vi "VIP Message.vi"(5 "Latest VIP":T1, 8 "Latest Version":string, 9 "Current Version":string) -> (3 "Continue":bool)   [LabVIEW 2014, in "Raspberry Pi Compatible Compiler for LabVIEW.lvlib"]
uses:
  Raspberry Pi Compatible Compiler for LabVIEW.lvlib
  System.Windows.Forms
  GitHub/TypeDefs/GitHubContents_TD.ctl
  Messaging/SimpleMessaging.lvlib
  GitHub/GitHub API.lvlib
panel:
  out "Animated Image":i16(ring) caption="Ring 2"
  out "Message":string
  in  "WebBrowser":refnum<k24>(container)
  in  "Compile":bool
  in  "Don't Continue":bool
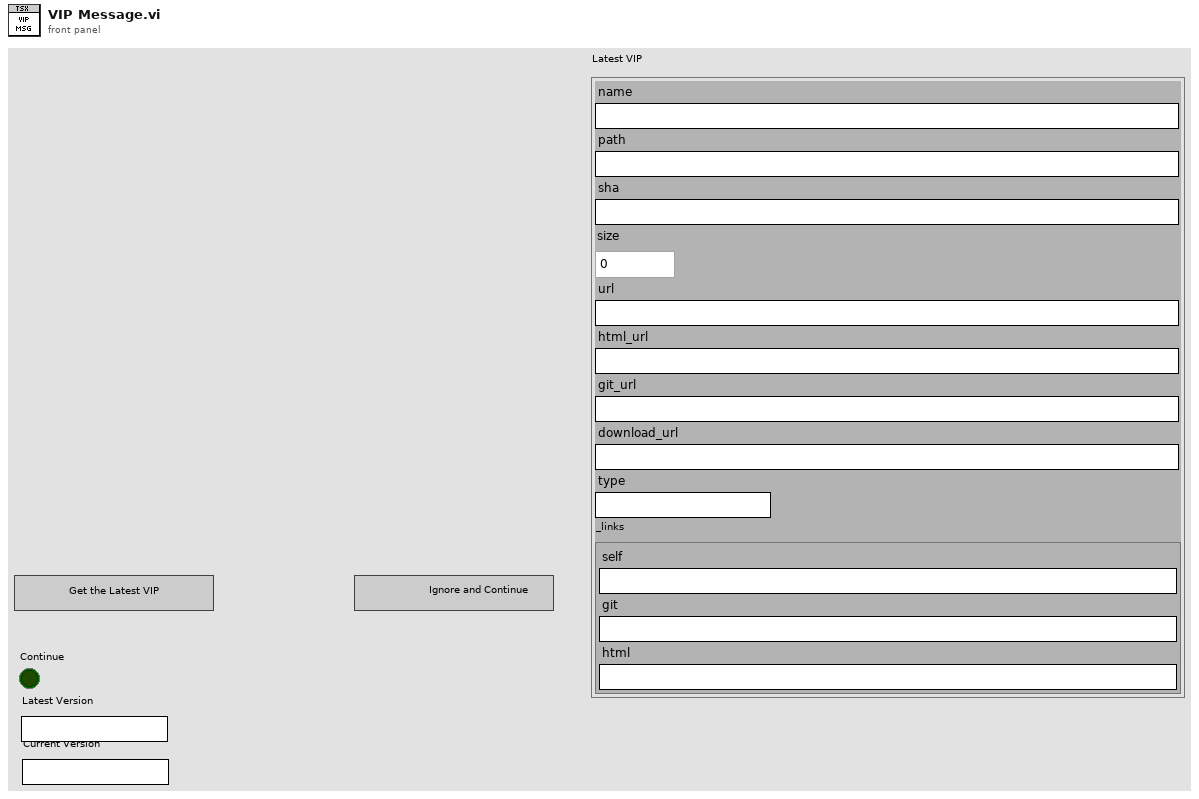
[diagram p1: front panel]
types:
  T1 = typedef "Raspberry Pi Compatible Compiler for LabVIEW.lvlib/GitHub API.lvlib/GitHubContents_TD.ctl" = cluster{"name":string, "path":string, "sha":string, "size":dbl, "url":string, "html_url":string, "git_url":string, "download_url":string, "type":string, "_links":cluster{"self":string, "git":string, "html":string}}
  T2 = typedef "Raspberry Pi Compatible Compiler for LabVIEW.lvlib/SimpleMessaging.lvlib/MessageQueueTD.ctl" = refnum<queue>
  T3 = enum32{"Invalid", "Standard", "Closed", "Hidden", "Minimized", "Maximized"}
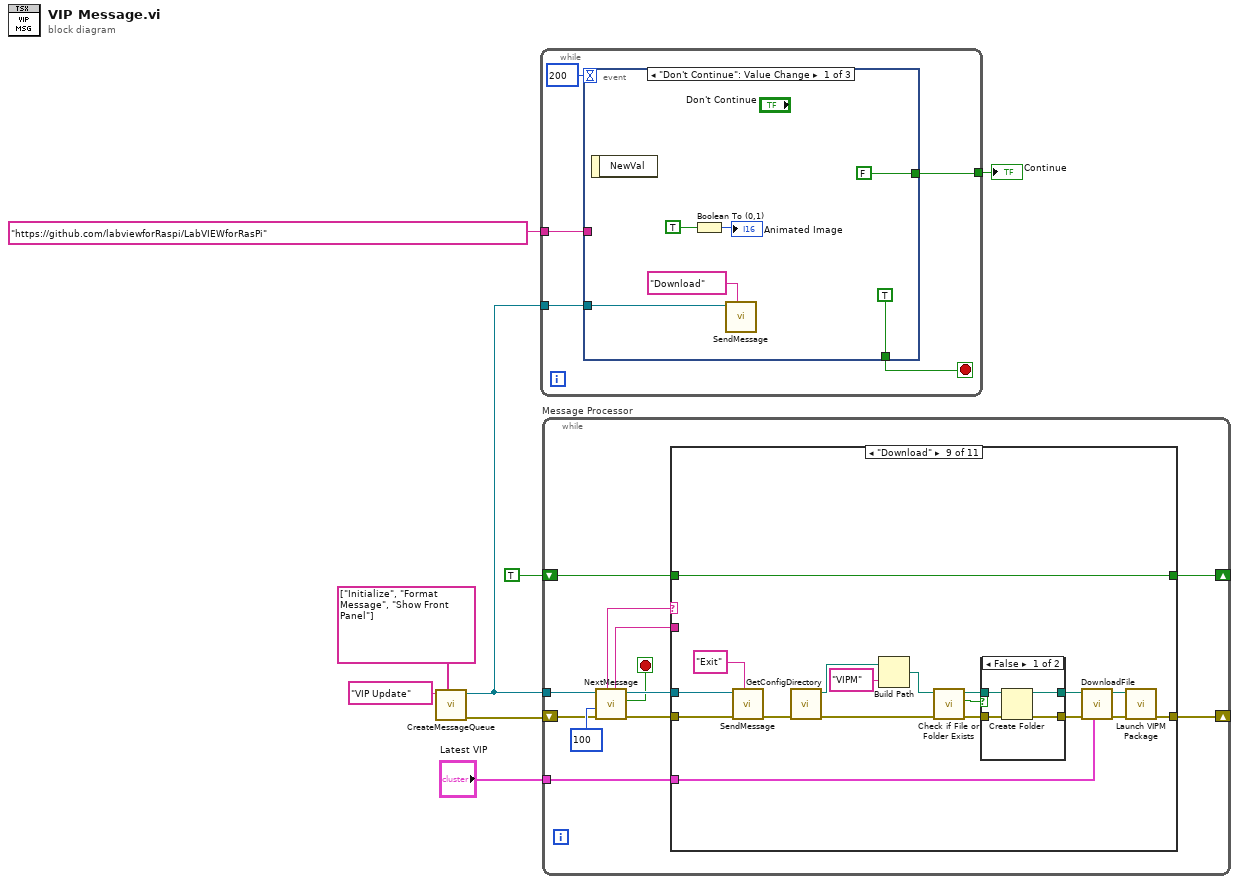
[diagram p0: block diagram]
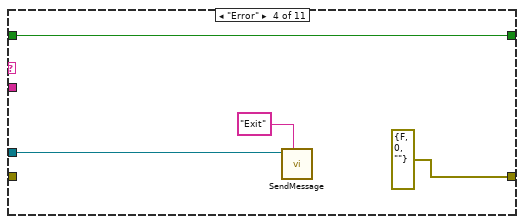
[diagram p5: hidden frame]
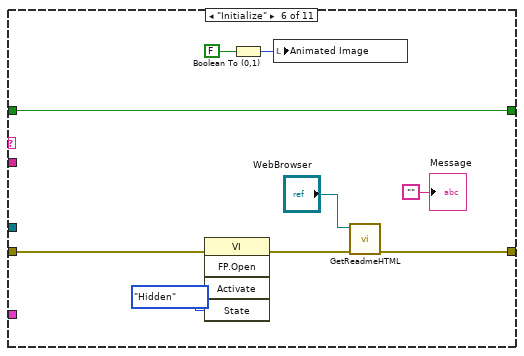
[diagram p7: hidden frame]
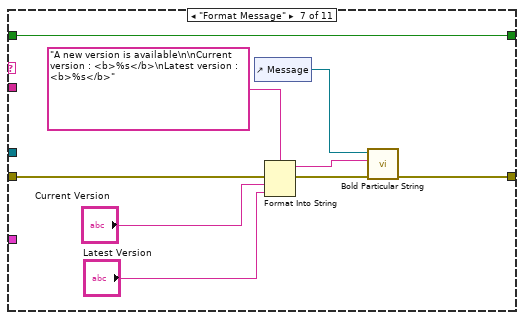
[diagram p8: hidden frame]
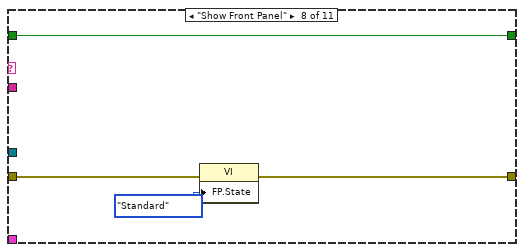
[diagram p9: hidden frame]
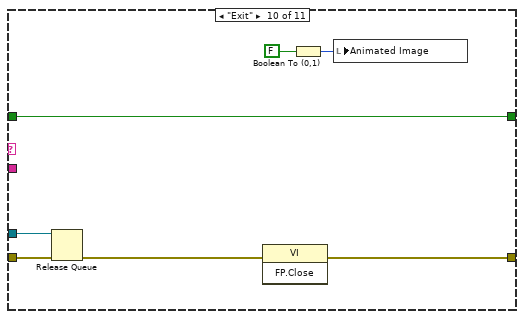
[diagram p11: hidden frame]
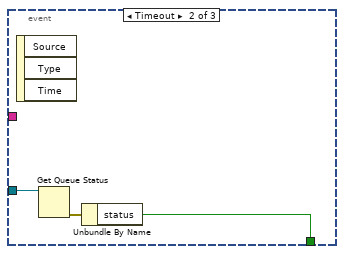
[diagram p13: hidden frame]
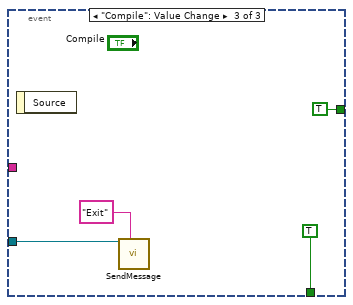
[diagram p14: hidden frame]
diagram:
  n1 = call "CreateMessageQueue.vi"("initial message names"=string[] ["Initialize", "Format Message", "Show Front Panel"], "message queue name"="VIP Update" ("name (unnamed)")) -> ("error out"=w2:errorcluster, "message queue out"=w3:T2)  [unwired: 5 in, 1 out]
  n2 = while {
    tunnel: "https://github.com/labviewforRaspi/LabVIEWforRasPi" ("URL") -> [w13]
    tunnel: [w12] -> w7
    tunnel: w3 -> [w10]
    stop <- w11 stop-if-true
    n3 = event shown="[0] \"Don't Continue\": Value Change" {
      selector: _ -> [_ _ _]
      dyn-events: _ -> [_ _ _]
      timeout: 200 -> [_ _ _]
      tunnel: w13 -> [_ _ _]
      tunnel: [TRUE w20 TRUE] -> w11
      tunnel: [FALSE _ TRUE] -> w12
      tunnel: w10 -> [w17 w22 w24]
      event "Don't Continue": Value Change {
        n4 = event-data() -> ()  [unwired: 1 in, 1 out]
        n5 = Boolean To (0,1)(Boolean=TRUE) -> (0, 1=→"Animated Image":i16)
        n6 = call "SendMessage.vi"("Name"="Download" ("Command"), "message queue in"=w17) -> ()  [unwired: 5 in, 3 out]
      }
      event Timeout {
        n7 = event-data() -> ()  [unwired: 1 in, 3 out]
        n8 = Get Queue Status(queue=w22) -> (error out=w21:errorcluster)  [unwired: 2 in, 7 out]
        n9 = Unbundle By Name(w21) -> ("status"=w20:bool)
      }
      event "Compile": Value Change {
        n10 = event-data() -> ()  [unwired: 1 in, 1 out]
        n11 = call "SendMessage.vi"("Name"="Exit", "message queue in"=w24) -> ()  [unwired: 5 in, 3 out]
      }
    }
  }
  "Continue" <- w7
  n12 = while "Message Processor" {
    shift-left: w2 -> [w29]
    shift-right: [w36] -> _
    shift-left: TRUE -> [w38]
    shift-right: [w37] -> _
    tunnel: w3 -> [w30]
    tunnel: "Latest VIP" -> [w27]
    stop <- w28 stop-if-true
    n13 = call "NextMessage.vi"("error in"=w29, "timeout in ms (-1)"=100 ("timeout in ms (100)"), "message queue in"=w30) -> ("error out"=w34:errorcluster, "exit"=w28:bool, "message queue out"=w31:T2, "Value"=w33:string, "Name"=w32:string)  [unwired: 1 in, 1 out]
    n14 = case shown="\"Download\"" w32 {
      tunnel: [w40 w42 w44 w48 w50 w59 w60 w71 w90 w103 w105] -> w37
      tunnel: w38 -> [w40 w42 w44 w48 w50 w59 w60 w71 w90 w103 w105]
      tunnel: w31 -> [_ _ _ w46 _ _ _ _ w76 w101 _]
      tunnel: w34 -> [w39 w41 w43 _ w49 w54 w64 w72 w78 w102 w104]
      tunnel: [w39 w41 w43 errorcluster {"status"=FALSE, "code"=0, "source"=""} ("error out") w49 w58 w67 w69 w73 w99 w104] -> w36
      tunnel: w33 -> [_ _ _ _ _ _ _ _ _ _ _]
      tunnel: w27 -> [_ _ _ _ _ _ _ _ w89 _ _]
      frame "---------- Framework Operations ----------" {
      }
      frame "", "Idle" {
      }
      frame Default {
      }
      frame "Error" {
        n15 = call "SendMessage.vi"("Name"="Exit" ("Command"), "message queue in"=w46) -> ()  [unwired: 5 in, 3 out]
      }
      frame "---------- Generic Operations ----------" {
      }
      frame "Initialize" {
        n16 = invoke class="VI" method="FP.Open"(error in=w54, "State"=T3."Hidden" ("Front Panel Window:State")) -> (error out=w53:errorcluster)  [unwired: 3 in, 4 out]
        n17 = Boolean To (0,1)(Boolean=FALSE) -> (0, 1=w51:i16)
        n18 = local write "Animated Image"(w51) -> ()
        n19 = call "GetReadmeHTML.vi"("error in"=w53, "WebBrowser in"="WebBrowser") -> ("error out"=w58:errorcluster)  [unwired: 6 in, 1 out]
        "Message" <- ""
      }
      frame "Format Message" {
        n20 = control-ref of="Message"() -> (w68:refnum<vi>)
        n21 = Format Into String(format string="A new version is available\n\nCurrent version : <b>%s</b>\nLatest version : <b>%s</b>" ("initial string"), error in=w64, "Current Version", "Latest Version") -> (resulting string=w66:string, error out=w65:errorcluster)  [unwired: 1 in]
        n22 = call <vilib>:"Bold Particular String.vi"("error in (no error)"=w65, "text to display"=w66, "string refnum"=w68) -> ("error out"=w67:errorcluster)  [unwired: 7 in, 1 out]
      }
      frame "Show Front Panel" {
        n23 = property class="VI"(error in=w72, "FP.State"=T3."Standard" ("Front Panel Window:State")) -> (error out=w69:errorcluster)  [unwired: 1 in, 1 out]
      }
      frame "Download" {
        n24 = call "SendMessage.vi"("Name"="Exit", "error in"=w78, "message queue in"=w76) -> ("error out"=w77:errorcluster)  [unwired: 4 in, 2 out]
        n25 = call "GetConfigDirectory.vi"("error in"=w77) -> ("error out"=w81:errorcluster, "config file directory out"=w88:path)  [unwired: 9 in]
        n26 = Build Path(base path=w88, name or relative path="VIPM") -> (appended path=w80:path)
        n27 = call <vilib>:"Check if File or Folder Exists.vi"("error in (no error)"=w81, "path"=w80) -> ("error out"=w86:errorcluster, "file or folder exists?"=w85:bool, "dup path"=w84:path)  [unwired: 7 in]
        n28 = case shown="False" w85 {
          tunnel: [w94 w96] -> w82
          tunnel: w84 -> [w93 w96]
          tunnel: w86 -> [w92 w95]
          tunnel: [w91 w95] -> w83
          frame False {
            n29 = Create Folder(path (use dialog)=w93, error in=w92) -> (created path=w94:path, error out=w91:errorcluster)  [unwired: 1 in, 1 out]
          }
          frame True {
          }
        }
        n30 = call "DownloadFile.vi"("Latest runtime"=w89, "error in"=w83, "Download Folder"=w82) -> ("error out"=w75:errorcluster, "file"=w74:path)  [unwired: 5 in]
        n31 = call "Launch VIPM Package.vi"("error in (no error)"=w75, "VIP File"=w74) -> ("error out"=w73:errorcluster)  [unwired: 9 in]
      }
      frame "Exit" {
        n32 = Release Queue(queue=w101, error in (no error)=w102) -> (error out=w100:errorcluster)  [unwired: 1 in, 2 out]
        n33 = invoke class="VI" method="FP.Close"(error in=w100) -> (error out=w99:errorcluster)  [unwired: 2 in, 2 out]
        n34 = Boolean To (0,1)(Boolean=FALSE) -> (0, 1=w97:i16)
        n35 = local write "Animated Image"(w97) -> ()
      }
      frame "---------- Application Operations ----------" {
      }
    }
  }
